vi "Hasmsg_2.vi"(8 "error in (no error)":errorcluster, 11 "OneOfTemplate in":refnum<class "w4lvgrpc_ToServer_payload.lvclass">) -> (0 "error out":errorcluster, 2 "Has Data?":bool, 3 "OneOfTemplate out":refnum<class "w4lvgrpc_ToServer_payload.lvclass">)   [LabVIEW 2019, in "Generated_server.lvlib" / "w4lvgrpc_ToServer_payload.lvclass"]
uses:
  w4lvgrpc_ToServer_payload.lvclass
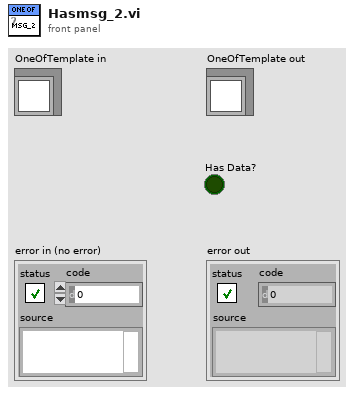
[diagram p1: front panel]
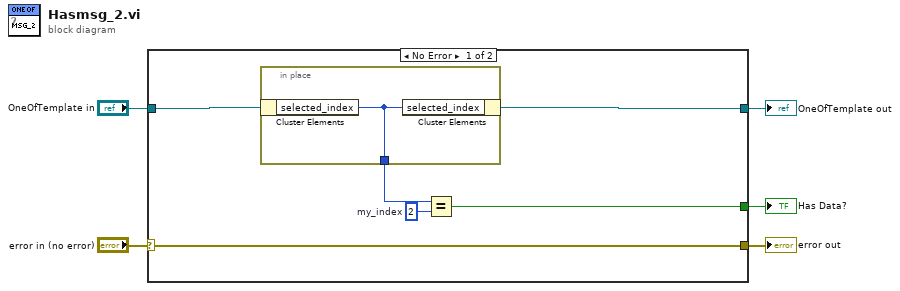
[diagram p0: block diagram]
diagram:
  n1 = case shown="No Error" "error in (no error)" {
    selector: "error in (no error)" -> [w11 w14]
    tunnel: [w11 w14] -> w4
    tunnel: [w7 w13] -> w2
    tunnel: "OneOfTemplate in" -> [w8 w13]
    tunnel: [w9 _] -> w1
    frame No Error {
      w10 = 2  # my_index
      n2 = in-place {
        in-place-border: [w12] -> w6
        n3 = in-place-cluster #1(w8) -> ("selected_index"=w12:i32)
        n4 = in-place-cluster #1("selected_index"=w12) -> (w7:refnum<class "w4lvgrpc_ToServer_payload.lvclass">)
      }
      n5 = Equal?(x=w6, y=w10) -> (x = y?=w9:bool)
    }
    frame Error {
    }
  }
  "error out" <- w4
  "OneOfTemplate out" <- w2
  "Has Data?" <- w1
